vi "TDMS Initialize.vi"(9 "Channel IDs":string[](array[string]), 10 "TDMS Name":string, 11 "Log to USB?":bool=TRUE) -> (3 "TDMS Cluster":T1)   [LabVIEW 2015]
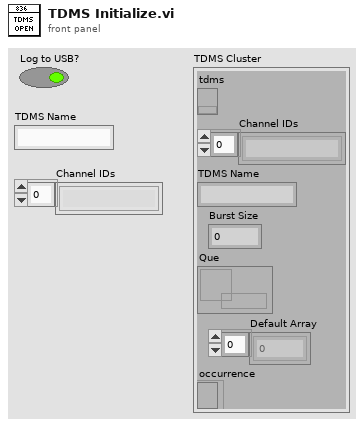
[diagram p1: front panel]
types:
  T1 = cluster{"tdms":refnum<k34>, "Channel IDs":string[], "TDMS Name":string, "Burst Size":i32, "Que":refnum<k33>, "Default Array":dbl[], "occurrence":refnum<k4>}
  T2 = enum16{"open", "open or create", "create or replace", "create", "open (read-only)"}
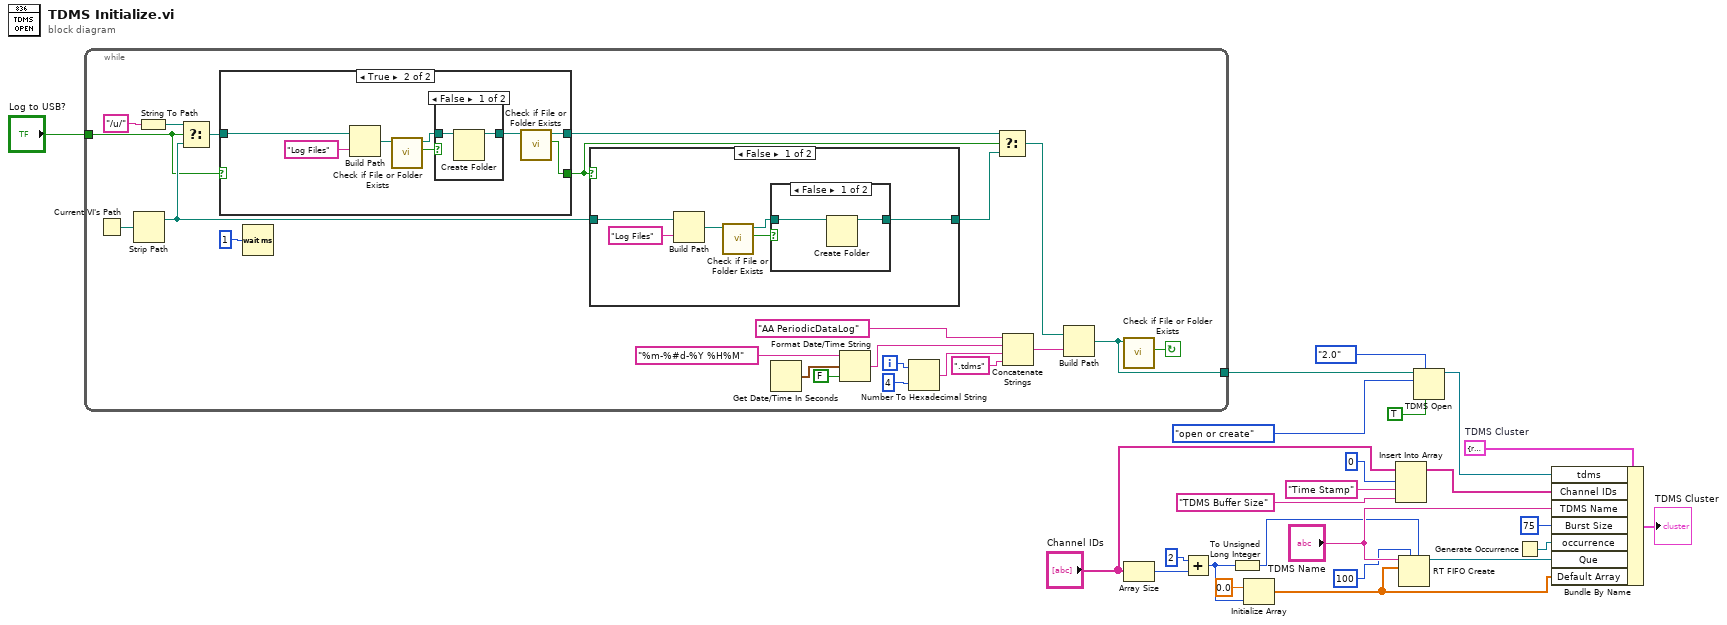
[diagram p0: block diagram]
diagram:
  w21 = T1 {"tdms"=refnum, "Channel IDs"=[], "TDMS Name"="", "Burst Size"=0, "Que"=refnum, "Default Array"=[], "occurrence"=refnum}  # TDMS Cluster
  n1 = while {
    tunnel: [w36] -> w11
    tunnel: "Log to USB?" -> [w25]
    i -> [w40]
    stop <- w37 continue-if-true
    n2 = Current VI's Path() -> (path=w35:path)
    n3 = Strip Path(path=w35) -> (stripped path=w29:path)  [unwired: 1 out]
    n4 = String To Path(string="/u/") -> (path=w33:path)
    n5 = Select(t=w33, s=w25, f=w29) -> (s? t:f=w34:path)
    n6 = case shown="True" w25 {
      selector: w25 -> [w49 _]
      tunnel: w34 -> [w48 w54]
      tunnel: [w48 w51] -> w31
      tunnel: [w49 w50] -> w28
      frame False {
      }
      frame True {
        n7 = Build Path(base path=w54, name or relative path="Log Files") -> (appended path=w53:path)
        n8 = call <vilib>:"Check if File or Folder Exists.vi"("path"=w53) -> ("file or folder exists?"=w57:bool, "dup path"=w56:path)  [unwired: 8 in, 1 out]
        n9 = case shown="False" w57 {
          tunnel: [w59 w60] -> w52
          tunnel: w56 -> [w58 w60]
          frame False {
            n10 = Create Folder(path (use dialog)=w58) -> (created path=w59:path)  [unwired: 2 in, 2 out]
          }
          frame True {
          }
        }
        n11 = call <vilib>:"Check if File or Folder Exists.vi"("path"=w52) -> ("file or folder exists?"=w50:bool, "dup path"=w51:path)  [unwired: 8 in, 1 out]
      }
    }
    n12 = Wait (ms)(milliseconds to wait=u32 1 ("millisecond multiple")) -> ()  [unwired: 1 out]
    n13 = case shown="False" w28 {
      tunnel: w29 -> [w65 w70]
      tunnel: [w61 w70] -> w27
      frame False {
        n14 = Build Path(base path=w65, name or relative path="Log Files") -> (appended path=w62:path)
        n15 = call <vilib>:"Check if File or Folder Exists.vi"("path"=w62) -> ("file or folder exists?"=w63:bool, "dup path"=w64:path)  [unwired: 8 in, 1 out]
        n16 = case shown="False" w63 {
          tunnel: [w68 w69] -> w61
          tunnel: w64 -> [w67 w69]
          frame False {
            n17 = Create Folder(path (use dialog)=w67) -> (created path=w68:path)  [unwired: 2 in, 2 out]
          }
          frame True {
          }
        }
      }
      frame True {
      }
    }
    n18 = Get Date/Time In Seconds() -> (seconds since 1Jan1904=w42:timestamp)
    n19 = Format Date/Time String(time format string (%c)="%m-%#d-%Y %H%M", seconds (now)=w42, UTC format=FALSE) -> (date/time string=w46:string)
    n20 = Number To Hexadecimal String(1:i16 4 ("width (-)"), 2:w40) -> (0:w38:string)
    n21 = Select(t=w31, s=w28, f=w27) -> (s? t:f=w30:path)
    n22 = Concatenate Strings("AA PeriodicDataLog" ("string"), w46, w38, ".tdms" ("string")) -> (w47:string)
    n23 = Build Path(base path=w30, name or relative path=w47) -> (appended path=w36:path)
    n24 = call <vilib>:"Check if File or Folder Exists.vi"("path"=w36) -> ("file or folder exists?"=w37:bool)  [unwired: 8 in, 2 out]
  }
  n25 = Array Size(array="Channel IDs") -> (size(s)=w10:i32)
  n26 = Add(x=2, y=w10) -> (x+y=w9:i32)
  n27 = To Unsigned Long Integer(number=w9) -> (unsigned 32bit integer=w8:u32)
  n28 = Initialize Array(0.0 ("element"), w9) -> (w17:dbl[])
  n29 = Insert Into Array(array="Channel IDs", index=0, new element #1="Time Stamp" ("new element/subarray"), new element #2="TDMS Buffer Size" ("new element/subarray")) -> (w1:string[])
  n30 = RT FIFO Create(0:"TDMS Name", 1:w17, 4:u32 100 ("size (10)"), 6:w8) -> (8:w18:refnum<k33>)  [unwired: 4 in, 2 out]
  n31 = TDMS Open(6:TRUE ("disable buffering? (T)"), 7:enum16{"1.0", "2.0"}."2.0" ("file format version (2.0)"), 10:T2."open or create" ("operation (0:open)"), 11:w11) -> (3:w20:refnum<k34>)  [unwired: 3 in, 1 out]
  n32 = Generate Occurrence() -> (w7:refnum<k4>)
  n33 = Bundle By Name(cluster=w21, "tdms"=w20, "Channel IDs"=w1, "TDMS Name"="TDMS Name", "Burst Size"=75 ("y"), "occurrence"=w7, "Que"=w18, "Default Array"=w17) -> (→"TDMS Cluster":T1)
